vi "ROI group interface-Temporary create ROI overlay.vi"(8 "error in":errorcluster, 9 "ROI X-Y data":i64[][](array[numeric]), 11 "Image In":T1) -> (0 "error out":errorcluster, 3 "Image Out":T1)   [LabVIEW 2020]
uses:
  <vilib>/vision/Image Controls.llb/IMAQ Image.ctl
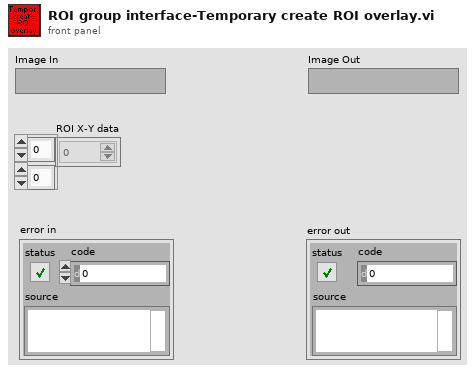
[diagram p1: front panel]
types:
  T1 = typedef "IMAQ Image.ctl" = refnum<image>
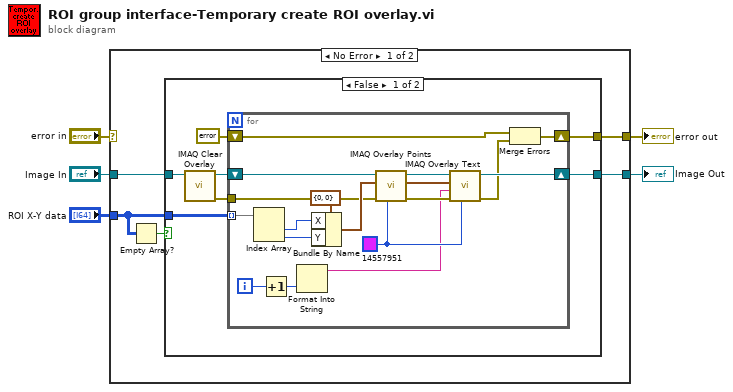
[diagram p0: block diagram]
diagram:
  n1 = case shown="No Error" "error in" {
    selector: "error in" -> [_ w36]
    tunnel: "Image In" -> [w6 w37]
    tunnel: "ROI X-Y data" -> [w10 _]
    tunnel: [w9 w37] -> w3
    tunnel: [w7 w36] -> w2
    frame No Error {
      n2 = Empty Array?(array=w10) -> (empty?=w8:bool)
      n3 = case shown="False" w8 {
        tunnel: w10 -> [w17 _]
        tunnel: w6 -> [w11 w35]
        tunnel: [w16 w35] -> w9
        tunnel: [w14 _] -> w7
        frame False {
          n4 = call "IMAQ Clear Overlay"("Image"=w11) -> ("error out"=w12:errorcluster, "Image Out"=w13:T1)  [unwired: 9 in]
          n5 = for {
            tunnel: w17 -> [w34] mode=indexing
            shift-right: [w22] -> w16
            shift-left: w13 -> [w23]
            tunnel: w12 -> [w21]
            shift-right: [w20] -> w14
            shift-left: errorcluster {"status"=FALSE, "code"=0, "source"=""} ("error IO") -> [w18]
            i -> [w26]
            w28 = u32 14557951 ("POI line Colour")
            n6 = Index Array(array=w34) -> (element #1=w31:i64, element #2=w30:i64)  [unwired: 2 in]
            n7 = Increment(x=w26) -> (x+1=w25:i32)
            n8 = Format Into String(w25) -> (resulting string=w24:string)  [unwired: 3 in, 1 out]
            n9 = Bundle By Name(cluster=cluster{"X":i32, "Y":i32} {"X"=0, "Y"=0} ("Point"), "X"=w31, "Y"=w30) -> (w27:cluster{"X":i32, "Y":i32})
            n10 = call "IMAQ Overlay Points"("Color"=w28, "error in (no error)"=w21, "Point"=w27, "Image"=w23) -> ("error out"=w33:errorcluster, "Image Out"=w32:T1)  [unwired: 6 in]
            n11 = call "IMAQ Overlay Text"("Text Color (black)"=w28, "error in (no error)"=w33, "String"=w24, "Origin"=w27, "Image"=w32) -> ("error out"=w19:errorcluster, "Image Out"=w22:T1)  [unwired: 5 in]
            n12 = Merge Errors(w18, w19) -> (w20:errorcluster)
          }
        }
        frame True {
          # "No POI data"
        }
      }
    }
    frame Error {
    }
  }
  "Image Out" <- w3
  "error out" <- w2
